vi "Read Voltage.vi"(0 "VISA resource name":refnum<visa-resource-name>, 11 "error in (no error)":errorcluster) -> (2 "Average Voltage":dbl, 3 "RMS Voltage":dbl, 4 "VISA resource name out":refnum<visa-resource-name>, 6 "High Voltage Level":dbl, 8 "Low Voltage Level":dbl, 13 "Maximum Voltage Level":dbl, 14 "Minimum Voltage Level":dbl, 15 "error out":errorcluster)   [LabVIEW 2019, in "Agilent N7976A.lvlib"]
doc: "Reads various voltage data. Responsible for triggering, waiting, and fetching the data."
uses:
  <instrlib>/Agilent N7976A/Agilent N7976A.lvlib
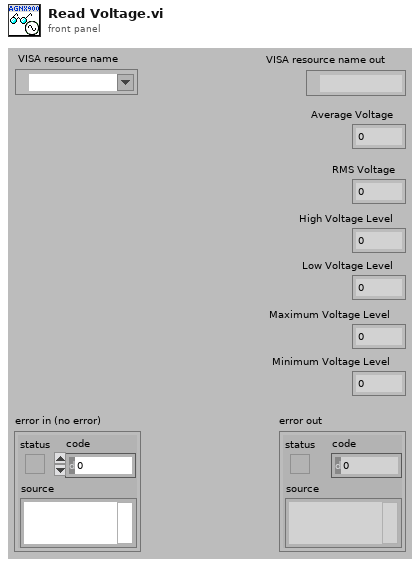
[diagram p1: front panel]
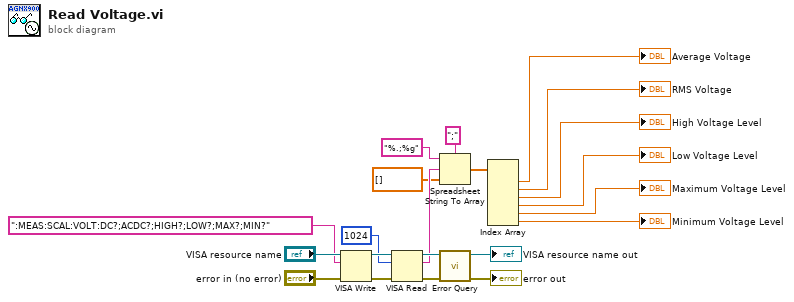
[diagram p0: block diagram]
diagram:
  n1 = VISA Write(VISA resource name="VISA resource name", write buffer=":MEAS:SCAL:VOLT:DC?;ACDC?;HIGH?;LOW?;MAX?;MIN?", error in (no error)="error in (no error)") -> (VISA resource name out=w16:refnum<visa-resource-name>, error out=w17:errorcluster)  [unwired: 1 out]
  n2 = VISA Read(VISA resource name=w16, byte count=u32 1024, error in (no error)=w17) -> (VISA resource name out=w18:refnum<visa-resource-name>, read buffer=w11:string, error out=w19:errorcluster)  [unwired: 1 out]
  n3 = Spreadsheet String To Array(delimiter (Tab)=";", format string="%.;%g", spreadsheet string=w11, array type (2D Dbl)=dbl[] []) -> (array=w8:dbl[])
  n4 = call <instrlib>:"Error Query.vi"("error in (no error)"=w19, "VISA resource name"=w18) -> ("error out"=→"error out":errorcluster, "VISA resource name out"=→"VISA resource name out":refnum<visa-resource-name>)  [unwired: 6 in, 2 out]
  n5 = Index Array(array=w8) -> (element #1=→"Average Voltage":dbl, element #2=→"RMS Voltage":dbl, element #3=→"High Voltage Level":dbl, element #4=→"Low Voltage Level":dbl, element #5=→"Maximum Voltage Level":dbl, element #6=→"Minimum Voltage Level":dbl)  [unwired: 6 in]
